vi "习3.2.vi"() -> ()   [LabVIEW 2017]
panel:
  out "数值 3":dbl
  in  "数值 2":dbl
  in  "数值":dbl
  in  "枚举":enum16{"相乘", "相除", "相加", "相减"}(ring)
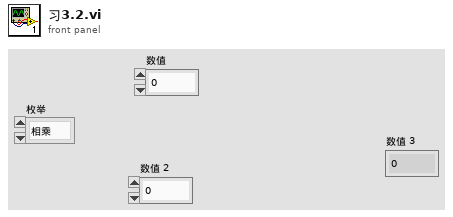
[diagram p1: front panel]
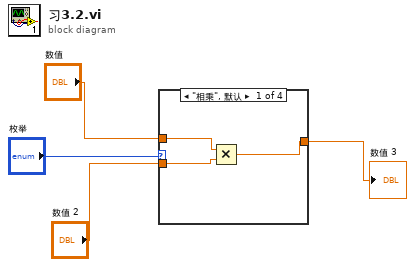
[diagram p0: block diagram]
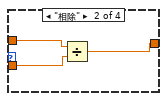
[diagram p2: hidden frame]
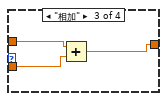
[diagram p3: hidden frame]
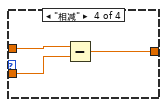
[diagram p4: hidden frame]
diagram:
  n1 = case shown="\"相乘\", 默认" "枚举" {
    tunnel: "数值 2" -> [w6 w8 w12 w16]
    tunnel: "数值" -> [w7 w9 w13 w15]
    tunnel: [w5 w10 w11 w14] -> w1
    frame "相乘", Default {
      n2 = Multiply(x=w7, y=w6) -> (x*y=w5:dbl)
    }
    frame "相除" {
      n3 = Divide(x=w9, y=w8) -> (x/y=w10:dbl)
    }
    frame "相加" {
      n4 = Add(x=w13, y=w12) -> (x+y=w11:dbl)
    }
    frame "相减" {
      n5 = Subtract(x=w15, y=w16) -> (x-y=w14:dbl)
    }
  }
  "数值 3" <- w1
